vi "Evaluate Macro_LOOPs.vi"(8 "Error In":errorcluster, 11 "Tree Refnum IN":refnum<vi>) -> (0 "Error Out":errorcluster, 2 "Macro Error":bool)   [LabVIEW 2012]
doc: "SciScan 1.2 160622"
uses:
  FGV_MacroCore_Commands.ctl
panel:
  out "Indices of Valid Items":i32[](array[numeric])
  out "x-y":u32
  out "Items":T1(array[cluster])
  out "Unbalanced LOOPs and Presets (Make red)":i32[](array[numeric])
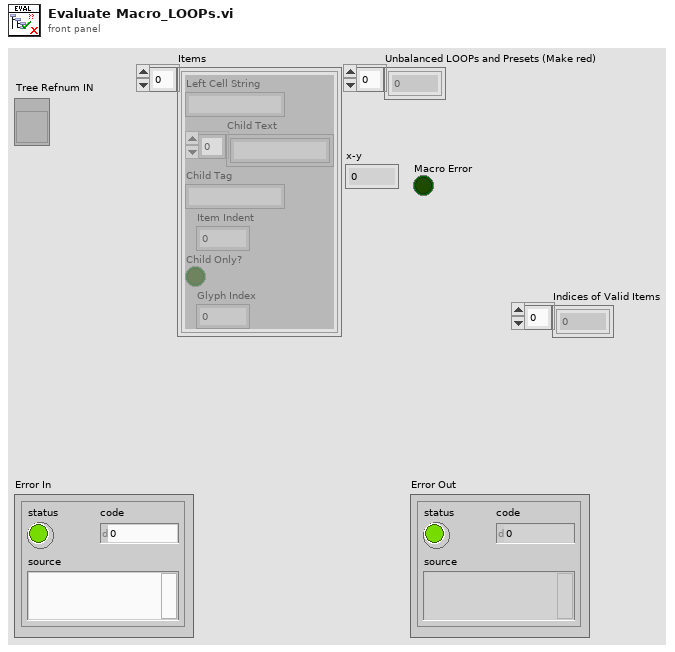
[diagram p1: front panel]
types:
  T1 = cluster{"Left Cell String":string, "Child Text":string[], "Child Tag":string, "Item Indent":i32, "Child Only?":bool, "Glyph Index":i32}[]
  T2 = typedef "FGV_MacroCore_Commands.ctl" = enum16{"Initialize", "Get Array", "Load macro from file", "Insert Item", "Insert at End", "Edit Parameter String", "Delete instruction", "Move Items", "Save", "SaveAs", "UpdateInfoTable", "Edit Settings File", "New Macro", "Read Temp File", "Delete Multiple"}
  T3 = cluster{"Left Cell String":string, "Child Text":string[], "Child Tag":string, "Item Indent":i32, "Child Only?":bool, "Glyph Index":i32}
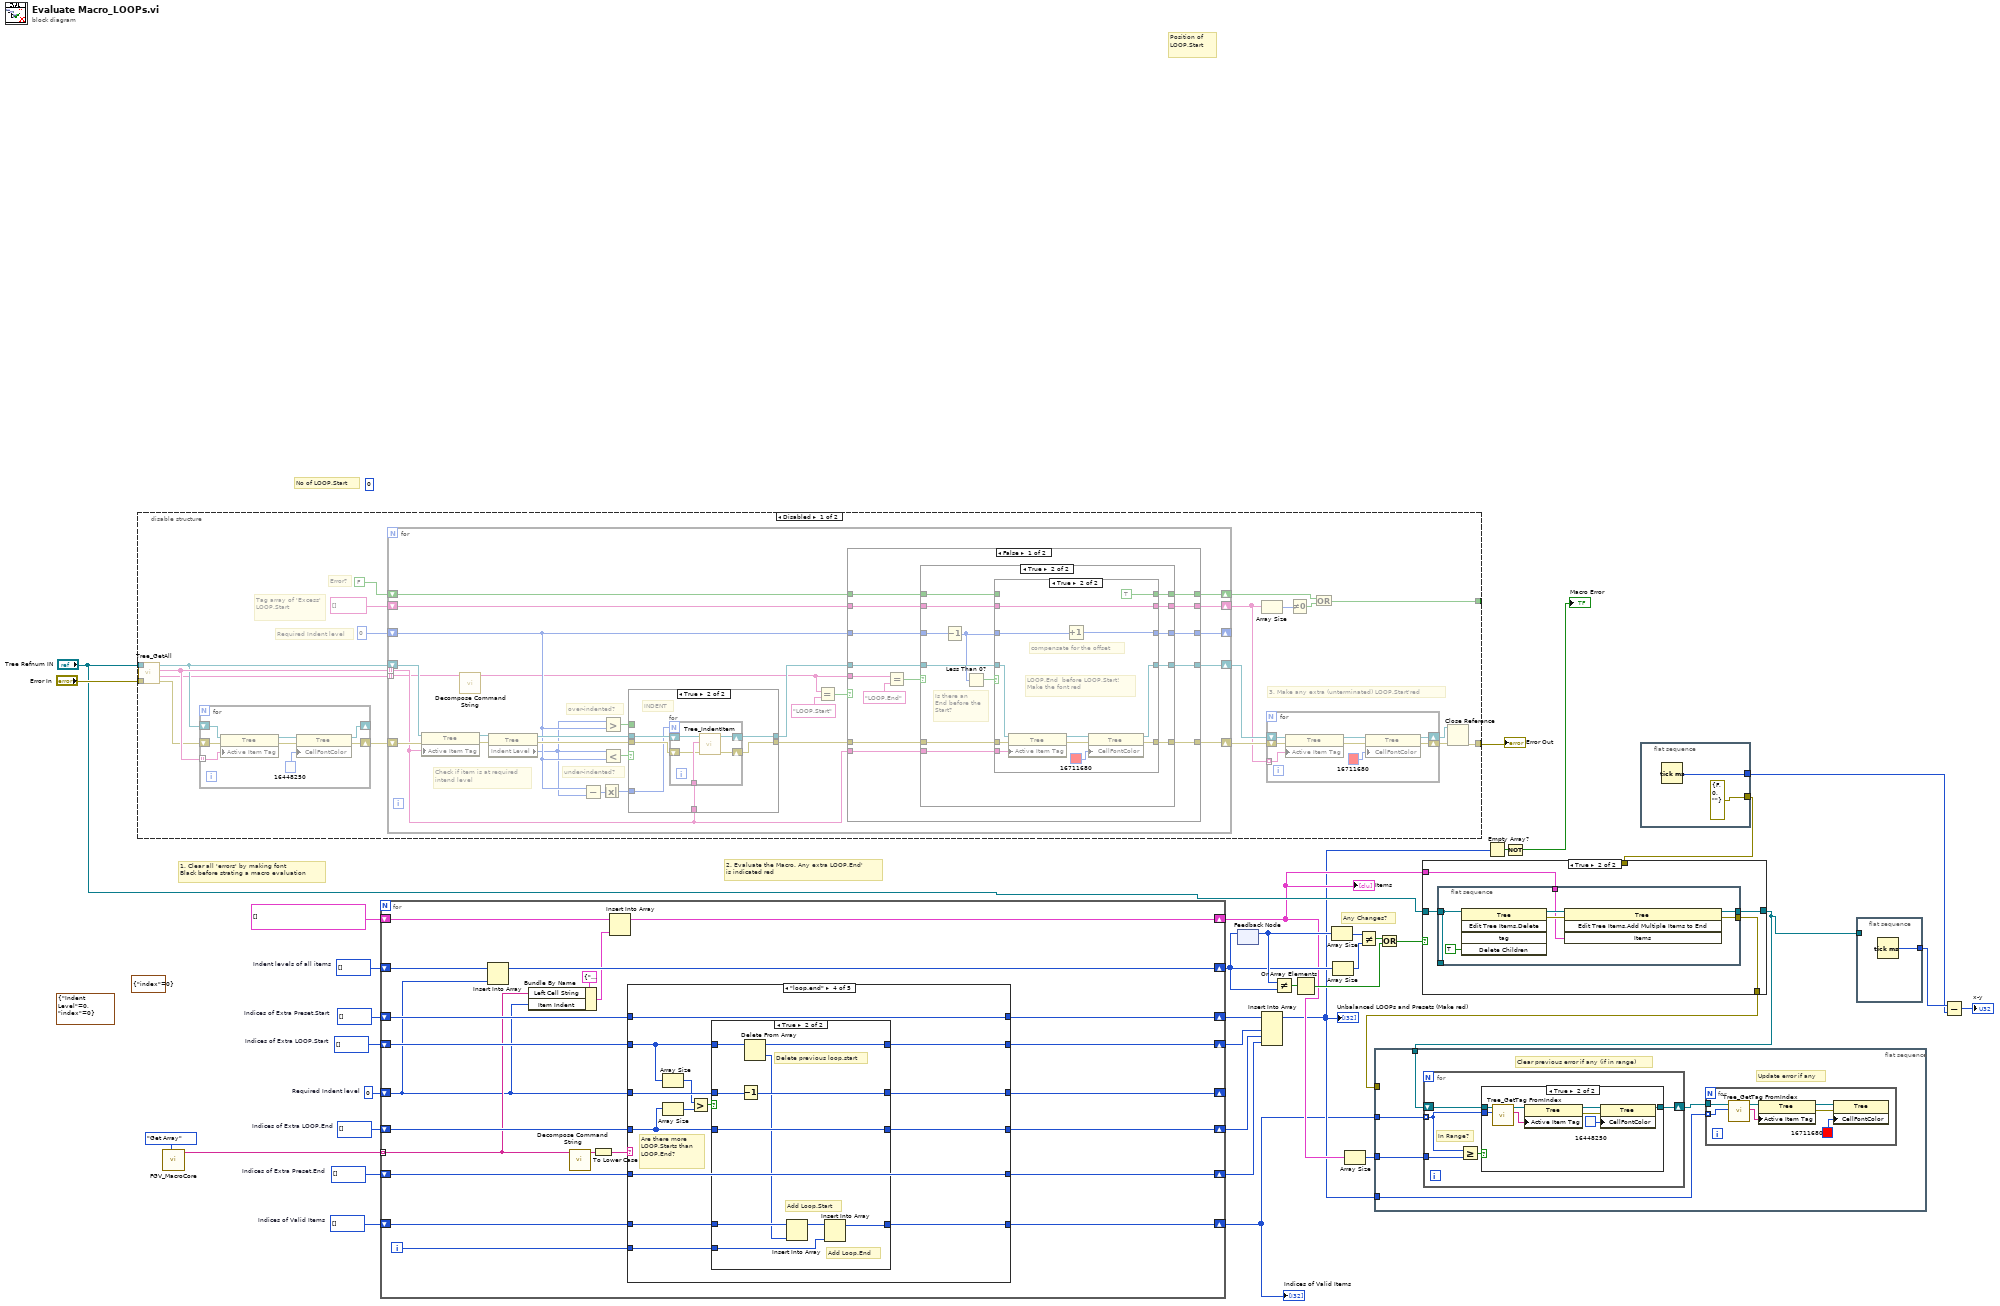
[diagram p0: block diagram]
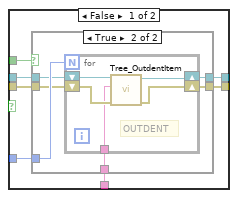
[diagram p2: hidden frame]
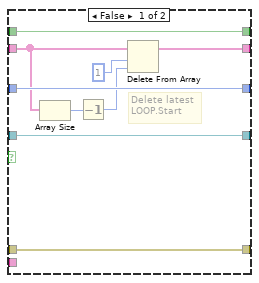
[diagram p5: hidden frame]
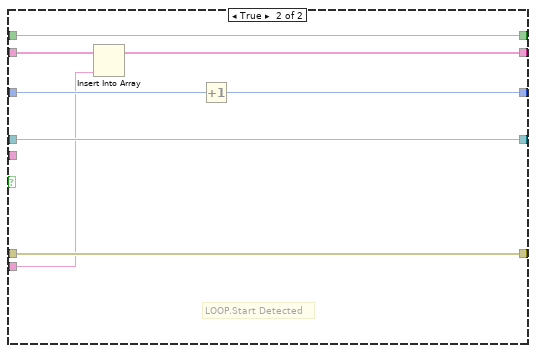
[diagram p6: hidden frame]
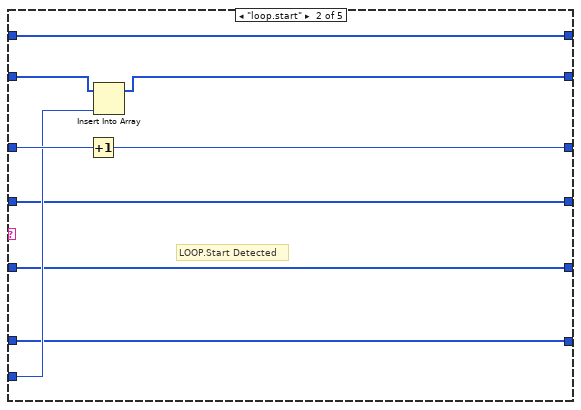
[diagram p11: hidden frame]
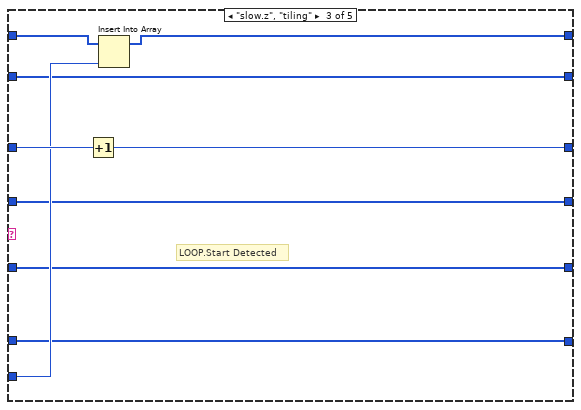
[diagram p12: hidden frame]
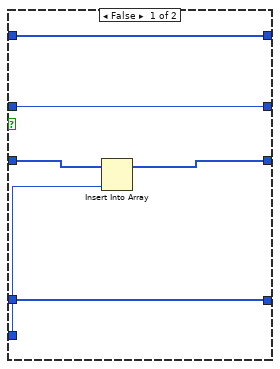
[diagram p13: hidden frame]
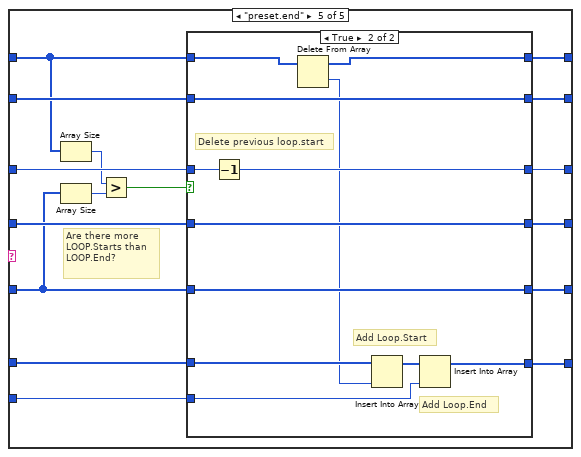
[diagram p14: hidden frame]
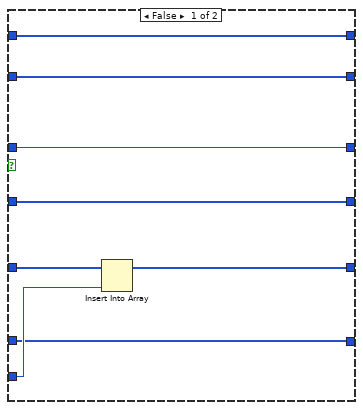
[diagram p15: hidden frame]
diagram:
  w2 = i32[] []  # Indices of Valid Items
  (unwired) cluster{"Indent Level":i32, "index":i32} {"Indent Level"=0, "index"=0}
  (unwired) cluster{"index":i32} {"index"=0}
  w28 = i32[] []  # Indices of Extra Preset.End
  w29 = i32[] []  # Indices of Extra Preset.Start
  w30 = i32[] []  # Indices of Extra LOOP.End
  w31 = i32[] []  # Indices of Extra LOOP.Start
  w32 = i32[] []  # Indent levels of all items
  w35 = 0  # Required Indent level
  (unwired) 0 ("index")
  # "Any Changes?"
  # "2. Evaluate the Macro. Any extra LOOP.End'\nis indicated red"
  # "1. Clear all 'errors' by making font\nBlack before strating a macro evaluation"
  # "No of LOOP.Start"
  # "Position of LOOP.Start"
  n1 = disable-structure shown="Disabled" {
    disable-tunnel: "Error In" -> [w56 _]
    disable-tunnel: [w44 _] -> _
    disable-tunnel: [w40 _] -> w36
    disable-tunnel: "Tree Refnum IN" -> [w38 _]
    frame Disabled {
      # "Error?"
      # "3. Make any extra (unterminated) LOOP.Start'red"
      # "Tag array of 'Excess' LOOP.Start"
      # "Required Indent level"
      n2 = call "Tree_GetAll.vi"("Error In"=w56, "Tree Refnum IN"=w38) -> ("Error Out"=w53:errorcluster, "Text"=w39:string[], "Tags"=w54:string[], "Tree Refnum OUT"=w52:refnum<vi>)  [unwired: 6 in]
      n3 = for {
        tunnel: w54 -> [w71] mode=indexing
        shift-right: [w68] -> w51
        shift-left: w53 -> [w73]
        shift-right: [w67] -> _
        shift-left: w52 -> [w72]
        n4 = property class="Tree"(reference=w72, error in=w73, "Active Item Tag"=w71) -> (reference out=w69:refnum<vi>, error out=w70:errorcluster)
        n5 = property class="Tree"(reference=w69, error in=w70, "CellFontColor"=u32 16448250) -> (reference out=w67:refnum<vi>, error out=w68:errorcluster)
      }
      n6 = for {
        tunnel: w39 -> [w75] mode=indexing
        shift-right: [w86] -> w50
        shift-left: w52 -> [w89]
        shift-right: [w90] -> _
        shift-left: 0 ("index") -> [w81]
        tunnel: w54 -> [w76] mode=indexing
        shift-right: [w85] -> w49
        shift-left: w51 -> [w82]
        shift-right: [w83] -> w48
        shift-left: string[] [] -> [w84]
        shift-right: [w78] -> w45
        shift-left: FALSE -> [w77]
        # "under-indented?"
        # "over-indented?"
        # "Check if item is at required\nintend level"
        n7 = property class="Tree"(reference=w89, error in=w82, "Active Item Tag"=w76) -> (reference out=w95:refnum<vi>, error out=w96:errorcluster)
        n8 = call "Decompose Command String.vi"("Command IN"=w75) -> ("Action"=w74:string)  [unwired: 7 in, 3 out]
        n9 = property class="Tree"(reference=w95, error in=w96) -> (reference out=w97:refnum<vi>, error out=w98:errorcluster, "Indent Level"=w80:i32)
        n10 = Subtract(x=w81, y=w80) -> (x-y=w92:i32)
        n11 = Absolute Value(x=w92) -> (abs(x)=w91:i32)
        n12 = Greater?(x=w80, y=w81) -> (0:w79:bool)
        n13 = Less?(x=w80, y=w81) -> (x < y?=w93:bool)
        n14 = case shown="True" w93 {
          tunnel: [w101 w125] -> w88
          tunnel: w76 -> [w102 w124]
          tunnel: [w100 w123] -> w87
          tunnel: w98 -> [w103 w122]
          tunnel: w97 -> [w104 w121]
          tunnel: w91 -> [w105 w120]
          tunnel: w79 -> [w106 _]
          frame False {
            n15 = case shown="True" w106 {
              tunnel: w105 -> [_ w114]
              tunnel: w104 -> [w108 w113]
              tunnel: w103 -> [w107 w112]
              tunnel: w102 -> [_ w111]
              tunnel: [w108 w110] -> w101
              tunnel: [w107 w109] -> w100
              frame False {
              }
              frame True {
                n16 = for {
                  N: w114 -> [_]
                  shift-right: [w116] -> w110
                  shift-left: w113 -> [w117]
                  shift-right: [w115] -> w109
                  shift-left: w112 -> [w119]
                  tunnel: w111 -> [w118]
                  # "OUTDENT"
                  n17 = call "Tree_OutdentItem.vi"("Error In"=w119, "TagToOutdent"=w118, "Tree Refnum"=w117) -> ("Error Out"=w115:errorcluster, "Tree Refnum OUT"=w116:refnum<vi>)  [unwired: 7 in]
                }
              }
            }
          }
          frame True {
            # "INDENT"
            n18 = for {
              N: w120 -> [_]
              tunnel: w124 -> [w129]
              shift-right: [w128] -> w123
              shift-left: w122 -> [w127]
              shift-right: [w130] -> w125
              shift-left: w121 -> [w126]
              n19 = call "Tree_IndentItem.vi"("Error In"=w127, "TagToIndent"=w129, "Tree Refnum"=w126) -> ("Error Out"=w128:errorcluster, "Tree Refnum OUT"=w130:refnum<vi>)  [unwired: 7 in]
            }
          }
        }
        n20 = Equal?(x=w74, y="LOOP.Start") -> (x = y?=w94:bool)
        n21 = case shown="False" w94 {
          tunnel: w88 -> [w139 w189]
          tunnel: w81 -> [w142 w191]
          tunnel: w74 -> [w143 _]
          tunnel: [w141 w190] -> w90
          tunnel: w76 -> [w140 w185]
          tunnel: [w138 w189] -> w86
          tunnel: w87 -> [w137 w188]
          tunnel: [w136 w188] -> w85
          tunnel: w84 -> [w134 w187]
          tunnel: [w133 w186] -> w83
          tunnel: [w132 w184] -> w78
          tunnel: w77 -> [w131 w184]
          frame False {
            n22 = Equal?(x=w143, y="LOOP.End") -> (x = y?=w135:bool)
            n23 = case shown="True" w135 {
              tunnel: w142 -> [w149 w155]
              tunnel: [w149 w162] -> w141
              tunnel: w140 -> [_ w161]
              tunnel: w139 -> [w148 w160]
              tunnel: [w148 w159] -> w138
              tunnel: w137 -> [w147 w158]
              tunnel: [w147 w157] -> w136
              tunnel: w134 -> [w146 w153]
              tunnel: [w146 w152] -> w133
              tunnel: [w145 w151] -> w132
              tunnel: w131 -> [w145 w150]
              frame False {
                # "Some other command\n- Do nothing"
              }
              frame True {
                # "Is there an \nEnd before the\nStart?"
                n24 = Decrement(x=w155) -> (x-1=w154:i32)
                n25 = Less Than 0?(x=w154) -> (x < 0?=w156:bool)
                n26 = case shown="True" w156 {
                  tunnel: w154 -> [w169 w174]
                  tunnel: [w169 w173] -> w162
                  tunnel: w161 -> [_ w183]
                  tunnel: w160 -> [w170 w179]
                  tunnel: [w170 w178] -> w159
                  tunnel: w158 -> [w171 w177]
                  tunnel: [w171 w176] -> w157
                  tunnel: w153 -> [w167 w175]
                  tunnel: [w168 w175] -> w152
                  tunnel: [w163 TRUE] -> w151
                  tunnel: w150 -> [w163 _]
                  frame False {
                    # "Delete latest LOOP.Start"
                    n27 = Array Size(array=w167) -> (size(s)=w166:i32)
                    n28 = Decrement(x=w166) -> (x-1=w164:i32)
                    n29 = Delete From Array(array=w167, length=1, index=w164) -> (array with subset deleted=w168:string[])  [unwired: 1 out]
                  }
                  frame True {
                    # "compensate for the offset"
                    # "LOOP.End  before LOOP.Start!\nMake the font red"
                    n30 = property class="Tree"(reference=w179, error in=w177, "Active Item Tag"=w183) -> (reference out=w182:refnum<vi>, error out=w181:errorcluster)
                    n31 = Increment(x=w174) -> (x+1=w173:i32)
                    n32 = property class="Tree"(reference=w182, error in=w181, "CellFontColor"=u32 16711680) -> (reference out=w178:refnum<vi>, error out=w176:errorcluster)
                  }
                }
              }
            }
          }
          frame True {
            # "LOOP.Start Detected"
            n33 = Insert Into Array(array=w187, new element=w185) -> (w186:string[])  [unwired: 1 in]
            n34 = Increment(x=w191) -> (x+1=w190:i32)
          }
        }
      }
      n35 = Array Size(array=w48) -> (size(s)=w47:i32)
      n36 = for {
        tunnel: w48 -> [w59] mode=indexing
        shift-right: [w60] -> w42
        shift-left: w49 -> [w61]
        shift-right: [w58] -> w41
        shift-left: w50 -> [w62]
        n37 = property class="Tree"(reference=w62, error in=w61, "Active Item Tag"=w59) -> (reference out=w63:refnum<vi>, error out=w64:errorcluster)
        n38 = property class="Tree"(reference=w63, error in=w64, "CellFontColor"=u32 16711680) -> (reference out=w58:refnum<vi>, error out=w60:errorcluster)
      }
      n39 = Not Equal To 0?(x=w47) -> (x != 0?=w46:bool)
      n40 = Or(x=w45, y=w46) -> (x .or. y?=w44:bool)
      n41 = Close Reference(reference=w41, error in (no error)=w42) -> (error out=w40:errorcluster)
    }
    frame Enabled {
    }
  }
  "Error Out" <- w36
  n42 = call "FGV_MacroCore.vi"("MacroFGV_Commands"=FGV_MacroCore_Commands."Get Array") -> ("Macro String Array"=w33:string[])  [unwired: 6 in, 4 out]
  n43 = for {
    tunnel: w33 -> [w196] mode=indexing
    shift-right: [w201] -> _
    shift-left: w35 -> [w194]
    shift-right: [w211] -> w13
    shift-left: w32 -> [w213]
    shift-right: [w210] -> w25
    shift-left: w31 -> [w212]
    shift-right: [w204] -> w26
    shift-left: w30 -> [w207]
    shift-right: [w205] -> w27
    shift-left: w29 -> [w208]
    shift-right: [w203] -> w8
    shift-left: w28 -> [w206]
    shift-right: [w197] -> w11
    shift-left: T1 [] ("Items") -> [w199]
    shift-right: [w192] -> w1
    shift-left: w2 -> [w193]
    i -> [w202]
    n44 = Insert Into Array(array=w213, new element=w194) -> (w211:i32[])  [unwired: 1 in]
    n45 = Bundle By Name(cluster=T3 {"Left Cell String"="", "Child Text"=[], "Child Tag"="", "Item Indent"=0, "Child Only?"=FALSE, "Glyph Index"=0} ("Item"), "Left Cell String"=w196, "Item Indent"=w194) -> (w198:T3)
    n46 = call "Decompose Command String.vi"("Command IN"=w196) -> ("Action"=w195:string)  [unwired: 7 in, 3 out]
    n47 = To Lower Case(string=w195) -> (all lower case string=w209:string)
    n48 = Insert Into Array(array=w199, new element=w198) -> (w197:T1)  [unwired: 1 in]
    n49 = case shown="\"loop.end\"" w209 {
      tunnel: w194 -> [w217 w228 w237 w251 w283]
      tunnel: [w217 w227 w236 w250 w282] -> w201
      tunnel: w212 -> [w218 w226 w231 w246 w280]
      tunnel: [w218 w224 w231 w249 w281] -> w210
      tunnel: w208 -> [w219 w223 w232 w248 w273]
      tunnel: w207 -> [w216 w222 w234 w242 w276]
      tunnel: w206 -> [w215 w221 w233 w247 w270]
      tunnel: w202 -> [_ w225 w235 w240 w274]
      tunnel: [w219 w223 w230 w248 w272] -> w205
      tunnel: [w216 w222 w234 w241 w275] -> w204
      tunnel: [w215 w221 w233 w247 w271] -> w203
      tunnel: w193 -> [w214 w220 w229 w239 w269]
      tunnel: [w214 w220 w229 w238 w268] -> w192
      frame Default {
        # "Some other command"
      }
      frame "loop.start" {
        # "LOOP.Start Detected"
        n50 = Increment(x=w228) -> (x+1=w227:i32)
        n51 = Insert Into Array(array=w226, new element=w225) -> (w224:i32[])  [unwired: 1 in]
      }
      frame "slow.z", "tiling" {
        # "LOOP.Start Detected"
        n52 = Increment(x=w237) -> (x+1=w236:i32)
        n53 = Insert Into Array(array=w232, new element=w235) -> (w230:i32[])  [unwired: 1 in]
      }
      frame "loop.end" {
        # "Are there more LOOP.Starts than LOOP.End?"
        n54 = Array Size(array=w246) -> (size(s)=w245:i32)
        n55 = Array Size(array=w242) -> (size(s)=w244:i32)
        n56 = Greater?(x=w245, y=w244) -> (0:w243:bool)
        n57 = case shown="True" w243 {
          tunnel: w251 -> [w256 w267]
          tunnel: [w256 w266] -> w250
          tunnel: [w257 w265] -> w249
          tunnel: w246 -> [w257 w264]
          tunnel: w242 -> [w255 w263]
          tunnel: [w254 w263] -> w241
          tunnel: w240 -> [w253 w259]
          tunnel: w239 -> [w252 w262]
          tunnel: [w252 w258] -> w238
          frame False {
            n58 = Insert Into Array(array=w255, new element=w253) -> (w254:i32[])  [unwired: 1 in]
          }
          frame True {
            # "Add Loop.End"
            # "Add Loop.Start"
            # "Delete previous loop.start"
            n59 = Decrement(x=w267) -> (x-1=w266:i32)
            n60 = Delete From Array(array=w264) -> (deleted portion=w261:i32, array with subset deleted=w265:i32[])  [unwired: 2 in]
            n61 = Insert Into Array(array=w262, new element=w261) -> (w260:i32[])  [unwired: 1 in]
            n62 = Insert Into Array(array=w260, new element=w259) -> (w258:i32[])  [unwired: 1 in]
          }
        }
      }
      frame "preset.end" {
        # "Are there more LOOP.Starts than LOOP.End?"
        n63 = Array Size(array=w273) -> (size(s)=w279:i32)
        n64 = Array Size(array=w270) -> (size(s)=w278:i32)
        n65 = Greater?(x=w279, y=w278) -> (0:w277:bool)
        n66 = case shown="True" w277 {
          tunnel: w283 -> [w290 w303]
          tunnel: [w290 w302] -> w282
          tunnel: [w291 w298] -> w281
          tunnel: w280 -> [w291 w298]
          tunnel: w276 -> [w286 w301]
          tunnel: [w286 w301] -> w275
          tunnel: w274 -> [w289 w292]
          tunnel: w273 -> [w285 w300]
          tunnel: [w285 w299] -> w272
          tunnel: [w287 w297] -> w271
          tunnel: w270 -> [w288 w297]
          tunnel: w269 -> [w284 w295]
          tunnel: [w284 w293] -> w268
          frame False {
            n67 = Insert Into Array(array=w288, new element=w289) -> (w287:i32[])  [unwired: 1 in]
          }
          frame True {
            # "Add Loop.End"
            # "Add Loop.Start"
            # "Delete previous loop.start"
            n68 = Decrement(x=w303) -> (x-1=w302:i32)
            n69 = Delete From Array(array=w300) -> (deleted portion=w294:i32, array with subset deleted=w299:i32[])  [unwired: 2 in]
            n70 = Insert Into Array(array=w295, new element=w294) -> (w296:i32[])  [unwired: 1 in]
            n71 = Insert Into Array(array=w296, new element=w292) -> (w293:i32[])  [unwired: 1 in]
          }
        }
      }
    }
  }
  "Items" <- w11
  "Indices of Valid Items" <- w1
  n72 = feedback-in #1(w13) -> ()
  n73 = feedback #1() -> (w22:i32[])  [unwired: 1 in]
  n74 = Insert Into Array(array=w27, new element #1=w25, new element #2=w26, new element #3=w8) -> (w9:i32[])  [unwired: 1 in]
  "Unbalanced LOOPs and Presets (Make red)" <- w9
  n75 = Not Equal?(x=w22, y=w13) -> (x != y?=w23:bool[])
  n76 = Or Array Elements(Boolean array=w23) -> (logical OR=w18:bool)
  n77 = Array Size(array=w22) -> (size(s)=w21:i32)
  n78 = Array Size(array=w13) -> (size(s)=w20:i32)
  n79 = Array Size(array=w11) -> (size(s)=w10:i32)
  n80 = Not Equal?(x=w21, y=w20) -> (x != y?=w19:bool)
  n81 = flat-sequence {
    tunnel: w9 -> [w308]
    tunnel: w4 -> [w307]
    tunnel: w15 -> [_]
    tunnel: w10 -> [w306]
    tunnel: w1 -> [w304]
    frame #0 {
      # "Update error if any"
      # "Clear previous error if any (if in range)"
      n82 = for {
        tunnel: w304 -> [w316] mode=indexing
        tunnel: w306 -> [w319]
        shift-right: [w320] -> w305
        shift-left: w307 -> [w317]
        # "In Range?"
        n83 = Greater Or Equal?(x=w316, y=w319) -> (x >= y?=w318:bool)
        n84 = case shown="True" w318 {
          tunnel: w317 -> [w321 w324]
          tunnel: [w321 w326] -> w320
          tunnel: w316 -> [_ w322]
          frame False {
          }
          frame True {
            n85 = call "Tree_GetTag FromIndex.vi"("Index IN"=w322, "Tree Refnum IN"=w324) -> ("Tag OUT"=w325:string, "Tree Refnum OUT"=w323:refnum<vi>)  [unwired: 7 in, 1 out]
            n86 = property class="Tree"(reference=w323, "Active Item Tag"=w325) -> (reference out=w328:refnum<vi>, error out=w329:errorcluster)  [unwired: 1 in]
            n87 = property class="Tree"(reference=w328, error in=w329, "CellFontColor"=u32 16448250) -> (reference out=w326:refnum<vi>)  [unwired: 1 out]
          }
        }
      }
      n88 = for {
        tunnel: w308 -> [w312] mode=indexing
        tunnel: w305 -> [w313]
        n89 = call "Tree_GetTag FromIndex.vi"("Index IN"=w312, "Tree Refnum IN"=w313) -> ("Tag OUT"=w310:string, "Tree Refnum OUT"=w311:refnum<vi>)  [unwired: 7 in, 1 out]
        n90 = property class="Tree"(reference=w311, "Active Item Tag"=w310) -> (reference out=w314:refnum<vi>, error out=w315:errorcluster)  [unwired: 1 in]
        n91 = property class="Tree"(reference=w314, error in=w315, "CellFontColor"=u32 16711680) -> ()  [unwired: 2 out]
      }
    }
  }
  n92 = Or(x=w19, y=w18) -> (x .or. y?=w17:bool)
  n93 = case shown="True" w17 {
    tunnel: "Tree Refnum IN" -> [w330 w334]
    tunnel: w11 -> [_ w333]
    tunnel: [_ w332] -> w15
    tunnel: [w330 w331] -> w4
    tunnel: w3 -> [_ _]
    frame False {
    }
    frame True {
      n94 = flat-sequence {
        tunnel: [w337] -> _
        tunnel: w333 -> [w338]
        tunnel: w334 -> [w337]
        tunnel: [w336] -> w332
        tunnel: [w335] -> w331
        frame #0 {
          n95 = invoke class="Tree" method="Edit Tree Items.Delete"(reference=w337, "Delete Children"=TRUE ("Delete Children?")) -> (reference out=w340:refnum<vi>, error out=w339:errorcluster)  [unwired: 3 in, 3 out]
          n96 = invoke class="Tree" method="Edit Tree Items.Add Multiple Items to End"(reference=w340, error in=w339, "Items"=w338) -> (reference out=w335:refnum<vi>, error out=w336:errorcluster)  [unwired: 1 in, 2 out]
        }
      }
    }
  }
  n97 = Empty Array?(array=w9) -> (empty?=w14:bool)
  n98 = Not(x=w14) -> (.not. x?=→"Macro Error":bool)
  n99 = flat-sequence {
    tunnel: [w343] -> w5
    tunnel: [errorcluster {"status"=FALSE, "code"=0, "source"=""} ("error constant")] -> w3
    frame #0 {
      n100 = Tick Count (ms)() -> (millisecond timer value=w343:u32)
    }
  }
  n101 = flat-sequence {
    tunnel: [w344] -> w7
    tunnel: w4 -> [_]
    frame #0 {
      n102 = Tick Count (ms)() -> (millisecond timer value=w344:u32)
    }
  }
  n103 = Subtract(x=w7, y=w5) -> (x-y=→"x-y":u32)
